vi "E816_Sample_Application_1a.vi"() -> ()   [LabVIEW 2020]
doc: "This VI demonstrates how to initialize an E-816 system with more than one axis, how to move all connected axes and how to query for the position value. \n\nIn this example the E-816 is connected through USB. The Serial No. of the system to command is not known, so the \"Search for controllers\" control is left TRUE. The VI runs E816_Configuration_Setup.vi with specified settings, moves the connected axes relative to their current position, waits for the movement to finish and reads the position of the axes and the error status of the controller. Instead of calling the corresponding command VIs, it uses \"Split multiple axes command.vi\" which sends the chosen commands for the given axes one after another and returns the answer array (if any). The diagram shows how to combine the driver VIs for these tasks. \n\nFor an example of how to command a single axis E-816 system connected through RS-232 see E816_Sample_ Application_1.vi\n\nWarning: Before running this VI, modify the interface settings on the block diagram to reflect your configuration. The predefined settings provided with the VI probably do not match your system."
panel:
  in  "stop":bool
  in  "error in":errorcluster
  out "Running":bool caption="Configuration_Setup.vi is running"
  out "error out":errorcluster
  out "Position":dbl[](array[numeric]) format="%.6f"
  out "Conn. Axes":string[](array[string])
  out "Identification":string
  # "This VI demonstrates how to initialize an E-816 system with more than one axis, how to move all connected axes and how to query\nfor the position value. The VI runs E816_Configuration_Setup.vi with specified settings, moves the connected axes relative to their \ncurrent position and reads the position. Instead of calling the corresponding command VIs, it uses \"Split multiple axes command.vi\"\nwhich sends the chosen commands for the given axes one after another and returns the answer array (if any). The diagram shows\nhow to combine the driver VIs for these tasks. \n\nWarning: Before running this VI, modify the interface settings on the block diagram to reflect your configuration. The predefined \n                 settings provided with the VI probably do not match your system."
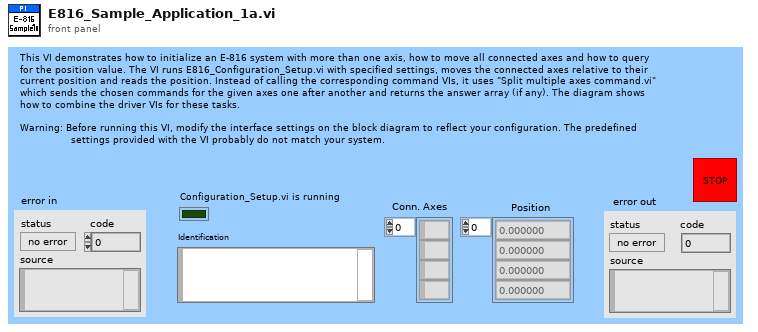
[diagram p1: front panel]
types:
  T1 = enum16{"DCO", "DCO?", "MOV", "MOV?", "MVR", "ONT?", "OVF?", "POS?", "RST", "SVA", "SVA?", "SVO", "SVO?", "SVR", "VOL?", "GWait"}
  T2 = enum16{"DCO", "DCO?", "MOV", "MOV?", "MVR", "ONT?", "OVF?", "POS?", "RST", "SVA", "SVA?", "SVO", "SVO?", "SVR", "VOL?"}
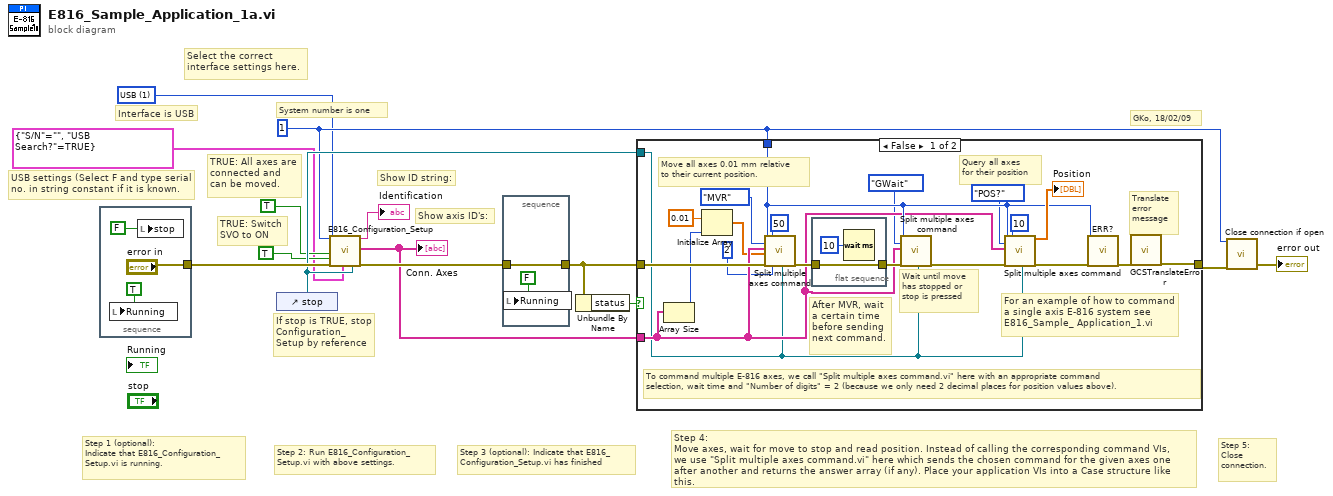
[diagram p0: block diagram]
diagram:
  w2 = u16 1 items=["RS232", "USB"] ("Interface")
  w3 = 1 ("System no.")
  # "USB settings (Select F and type serial\nno. in string constant if it is known."
  # "Interface is USB"
  # "Step 5: \nClose\nconnection."
  # "TRUE: All axes are\nconnected and\ncan be moved."
  # "TRUE: Switch\nSVO to ON"
  # "If stop is TRUE, stop\nConfiguration_\nSetup by reference"
  # "Step 4: \nMove axes, wait for move to stop and read position. Instead of calling the corresponding command VIs,\nwe use \"Split multiple axes command.vi\" here which sends the chosen command for the given axes one\nafter another and returns the answer array (if any). Place your application VIs into a Case structure like this."
  # "Select the correct\ninterface settings here."
  # "GKo, 18/02/09"
  # "Step 3 (optional): Indicate that E816_\nConfiguration_Setup.vi has finished"
  # "Step 2: Run E816_Configuration_\nSetup.vi with above settings."
  # "Step 1 (optional): \nIndicate that E816_Configuration_\nSetup.vi is running."
  # "Show axis ID's:"
  # "Show ID string:"
  # "System number is one"
  n1 = stacked-sequence {
    tunnel: ["error in"] -> w12
    frame #0 {
      n2 = local write "Running"(TRUE ("Running")) -> ()
      n3 = local write "stop"(FALSE ("stop")) -> ()
    }
  }
  n4 = control-ref of="stop"() -> (w8:refnum<vi>)
  n5 = call "E816_Configuration_Setup.vi"("System no."=w3, "Interface"=w2, "All axes?"=TRUE, "Change servo \nstatus to ON?"=TRUE ("Use dialog to define\nconnected stages?"), "error in"=w12, "USB settings"=cluster{"S/N":string, "USB Search?":bool} {"S/N"="", "USB Search?"=TRUE}, "Stop refnum"=w8) -> ("Identification"=→"Identification":string, "Conn. Axes"=w9:string[], "error out"=w13:errorcluster)  [unwired: 4 in, 6 out]
  "Conn. Axes" <- w9
  n6 = stacked-sequence {
    tunnel: w13 -> [w19]
    tunnel: [w19] -> w11
    frame #0 {
      n7 = local write "Running"(FALSE ("Running")) -> ()
    }
  }
  n8 = Unbundle By Name(w11) -> ("status"=w10:bool)
  n9 = case shown="False" w10 {
    tunnel: [w37 w42] -> w4
    tunnel: w9 -> [w30 _]
    tunnel: w3 -> [w34 _]
    tunnel: w11 -> [w38 w42]
    tunnel: w8 -> [w22 _]
    frame False {
      # "For an example of how to command\na single axis E-816 system see \nE816_Sample_ Application_1.vi"
      # "After MVR, wait\na certain time\nbefore sending\nnext command."
      # "Translate\nerror \nmessage"
      # "Wait until move\nhas stopped or\nstop is pressed"
      # "Query all axes\nfor their position"
      # "To command multiple E-816 axes, we call \"Split multiple axes command.vi\" here with an appropriate command\nselection, wait time and \"Number of digits\" = 2 (because we only need 2 decimal places for position values above)."
      # "Move all axes 0.01 mm relative\nto their current position."
      n10 = Array Size(array=w30) -> (size(s)=w29:i32)
      n11 = Initialize Array(0.01 ("Numeric"), w29) -> (w27:dbl[])
      n12 = call "Split multiple axes command.vi"("System no."=w34, "Command"=T2."MVR", "Axes to command"=w30, "Num. values in"=w27, "error in"=w38, "Wait time (ms)"=u32 50, "No.of digits"=i16 2, "Stop refnum"=w22) -> ("error out"=w32:errorcluster)  [unwired: 1 in, 10 out]
      n13 = flat-sequence {
        tunnel: w32 -> [w41]
        tunnel: [w41] -> w31
        frame #0 {
          n14 = Wait (ms)(milliseconds to wait=u32 10) -> ()  [unwired: 1 out]
        }
      }
      n15 = call "Split multiple axes command.vi"("System no."=w34, "Command"=T1."GWait", "Axes to command"=w30, "error in"=w31, "Stop refnum"=w22) -> ("error out"=w33:errorcluster)  [unwired: 4 in, 10 out]
      n16 = call "Split multiple axes command.vi"("System no."=w34, "Command"=T2."POS?", "Axes to command"=w30, "error in"=w33, "Wait time (ms)"=u32 10, "Stop refnum"=w22) -> ("Num. values out"=→"Position":dbl[], "error out"=w36:errorcluster)  [unwired: 3 in, 9 out]
      n17 = call "ERR?.vi"("System no."=w34, "error in"=w36) -> ("error out"=w35:errorcluster)  [unwired: 17 out]
      n18 = call "GCSTranslateError.vi"("error in"=w35) -> ("error out"=w37:errorcluster)  [unwired: 18 out]
    }
    frame True {
      # "Error during initialization"
    }
  }
  n19 = call "Close connection if open.vi"("System no."=w3, "error in"=w4) -> ("error out"=→"error out":errorcluster)  [unwired: 1 in, 16 out]
